vi "Obtain Session.vi"(6 "Debug Daemon (Dev Only)":bool, 8 "error in (no error)":errorcluster, 10 "Create if needed? (T)":bool=TRUE, 11 "TS License Type (Operator)":T1) -> (0 "error out":errorcluster, 3 "Engine out":refnum<class "Engine.lvclass">)   [LabVIEW 2020, in "TSnax.lvlib" / "Engine.lvclass"]
uses:
  Engine.lvclass
  TS License Type.ctl
  Engine.lvclass/Engine.ctl
  TSnax.lvlib
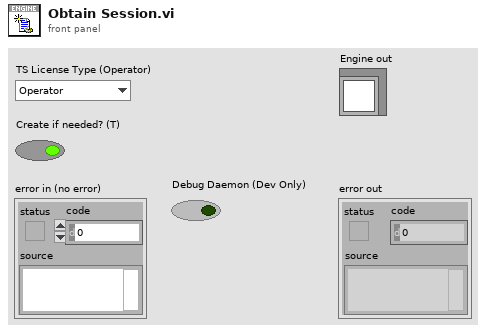
[diagram p1: front panel]
types:
  T1 = typedef "TSnax.lvlib/TS License Type.ctl" = enum16{"Operator", "CustomEditor", "SequenceEditor"}
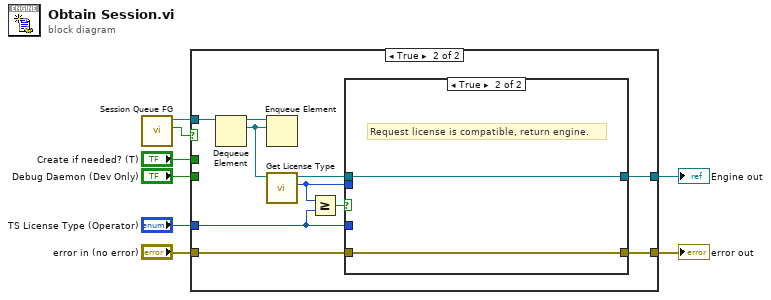
[diagram p0: block diagram]
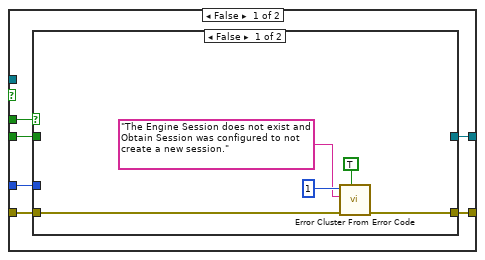
[diagram p2: hidden frame]
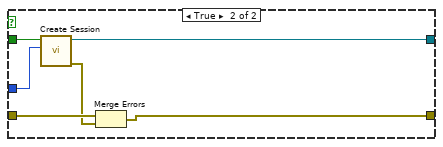
[diagram p3: hidden frame]
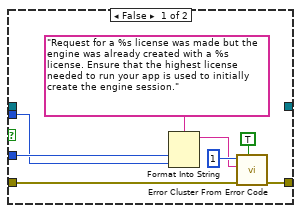
[diagram p4: hidden frame]
diagram:
  n1 = call "Session Queue FG.vi"() -> ("Session Valid?"=w7:bool, "Session Queue"=w6:refnum<queue>)  [unwired: 10 in]
  n2 = case shown="True" w7 {
    tunnel: "error in (no error)" -> [w12 w29]
    tunnel: w6 -> [_ w35]
    tunnel: "Create if needed? (T)" -> [w14 _]
    tunnel: "Debug Daemon (Dev Only)" -> [w9 _]
    tunnel: "TS License Type (Operator)" -> [w13 w28]
    tunnel: [w11 w30] -> w2
    tunnel: [w10 w26] -> w1
    frame False {
      n3 = case shown="False" w14 {
        tunnel: w13 -> [_ w20]
        tunnel: w12 -> [w19 w24]
        tunnel: [_ w25] -> w11
        tunnel: [w17 w22] -> w10
        tunnel: w9 -> [_ w21]
        frame False {
          n4 = call <vilib>:"Error Cluster From Error Code.vi"("show call chain? (False)"=TRUE, "error in (no error)"=w19, "error message (\"\")"="The Engine Session does not exist and Obtain Session was configured to not create a new session.", "error code (0)"=1) -> ("error out"=w17:errorcluster)  [unwired: 5 in]
        }
        frame True {
          n5 = call "Create Session.vi"("TS License Type"=w20, "Dev Debug?"=w21) -> ("error out"=w23:errorcluster, "Engine out"=w25:refnum<class "Engine.lvclass">)  [unwired: 8 in]
          n6 = Merge Errors(w24, w23) -> (w22:errorcluster)
        }
      }
    }
    frame True {
      n7 = Dequeue Element(queue=w35) -> (queue out=w34:refnum<queue>, element=w33:refnum<class "Engine.lvclass">)  [unwired: 2 in, 2 out]
      n8 = Enqueue Element(queue=w34, element=w33) -> ()  [unwired: 2 in, 3 out]
      n9 = call "Get License Type.vi"("Engine in"=w33) -> ("TS License Type"=w27:T1, "Engine out"=w31:refnum<class "Engine.lvclass">)  [unwired: 8 in, 1 out]
      n10 = Greater Or Equal?(x=w27, y=w28) -> (x >= y?=w32:bool)
      n11 = case shown="True" w32 {
        tunnel: w31 -> [_ w45]
        tunnel: [_ w45] -> w30
        tunnel: w29 -> [w43 w44]
        tunnel: w28 -> [w39 _]
        tunnel: w27 -> [w38 _]
        tunnel: [w36 w44] -> w26
        frame False {
          n12 = Format Into String(format string="Request for a %s license was made but the engine was already created with a %s license. Ensure that the highest license needed to run your app is used to initially create the engine session.", w39, w38) -> (resulting string=w37:string)  [unwired: 2 in, 1 out]
          n13 = call <vilib>:"Error Cluster From Error Code.vi"("show call chain? (False)"=TRUE, "error in (no error)"=w43, "error message (\"\")"=w37, "error code (0)"=1) -> ("error out"=w36:errorcluster)  [unwired: 5 in]
        }
        frame True {
          # "Request license is compatible, return engine."
        }
      }
    }
  }
  "error out" <- w1
  "Engine out" <- w2
